vi "map to well (ROI) simple.vi"(7 "centroids in":u16[][](array[numeric])=[[65535, 65535], [65535, 65535], [57, 304], [65535, 65535], [65535, 65535], [65535, 65535], [65535, 65535], [84, 793], [150, 86], [65535, 65535], [65535, 65535], [65535, 65535], [65535, 65535], [65535, 65535], [65535, 65535], [65535, 65535], [295, 112], [65535, 65535], [65535, 65535], [65535, 65535], [65535, 65535], [65535, 65535], [65535, 65535], [313, 848], [402, 114], [65535, 65535], [65535, 65535], [65535, 65535], [65535, 65535], [65535, 65535], [65535, 65535], [65535, 65535], [65535, 65535], [65535, 65535], [65535, 65535], [65535, 65535], [65535, 65535], [65535, 65535], [65535, 65535], [65535, 65535], [65535, 65535], [65535, 65535], [65535, 65535], [65535, 65535], [65535, 65535], [65535, 65535], [562, 690], [613, 846], [733, 113], [65535, 65535], [65535, 65535], [65535, 65535], [65535, 65535], [65535, 65535], [65535, 65535], [65535, 65535], [843, 133], [65535, 65535], [65535, 65535], [65535, 65535], [65535, 65535], [65535, 65535], [65535, 65535], [65535, 65535], [880, 72], [65535, 65535], [65535, 65535], [881, 382], [65535, 65535], [65535, 65535], [65535, 65535], [65535, 65535], [989, 67], [65535, 65535], [65535, 65535], [65535, 65535], [65535, 65535], [65535, 65535], [65535, 65535], [1004, 856], [65535, 65535], [1089, 232], [65535, 65535], [65535, 65535], [65535, 65535], [65535, 65535], [65535, 65535], [1100, 861], [1253, 78], [65535, 65535], [65535, 65535], [65535, 65535], [65535, 65535], [65535, 65535], [65535, 65535], [65535, 65535]], 10 "roi data cluster":T1={[0, 0, 1280, 960], [{"Contour Type"=0, "ROI Type"=12, [70, 141, 164, 235, 270302]}, {"Contour Type"=0, "ROI Type"=12, [70, 236, 164, 330, 270302]}, {"Contour Type"=0, "ROI Type"=12, [71, 331, 165, 425, 270302]}, {"Contour Type"=0, "ROI Type"=12, [72, 426, 166, 520, 270302]}, {"Contour Type"=0, "ROI Type"=12, [72, 520, 166, 614, 270302]}, {"Contour Type"=0, "ROI Type"=12, [72, 615, 166, 709, 270302]}, {"Contour Type"=0, "ROI Type"=12, [73, 710, 167, 804, 270302]}, {"Contour Type"=0, "ROI Type"=12, [74, 805, 168, 899, 270302]}, {"Contour Type"=0, "ROI Type"=12, [165, 140, 259, 234, 270302]}, {"Contour Type"=0, "ROI Type"=12, [165, 235, 259, 329, 270302]}, {"Contour Type"=0, "ROI Type"=12, [166, 330, 260, 424, 270302]}, {"Contour Type"=0, "ROI Type"=12, [166, 425, 260, 519, 270302]}, {"Contour Type"=0, "ROI Type"=12, [167, 520, 261, 614, 270302]}, {"Contour Type"=0, "ROI Type"=12, [167, 615, 261, 709, 270302]}, {"Contour Type"=0, "ROI Type"=12, [168, 710, 262, 804, 270302]}, {"Contour Type"=0, "ROI Type"=12, [168, 805, 262, 899, 270302]}, {"Contour Type"=0, "ROI Type"=12, [260, 140, 354, 234, 270302]}, {"Contour Type"=0, "ROI Type"=12, [260, 235, 354, 329, 270302]}, {"Contour Type"=0, "ROI Type"=12, [260, 330, 354, 424, 270302]}, {"Contour Type"=0, "ROI Type"=12, [261, 425, 355, 519, 270302]}, {"Contour Type"=0, "ROI Type"=12, [262, 520, 356, 614, 270302]}, {"Contour Type"=0, "ROI Type"=12, [262, 614, 356, 708, 270302]}, {"Contour Type"=0, "ROI Type"=12, [262, 709, 356, 803, 270302]}, {"Contour Type"=0, "ROI Type"=12, [263, 804, 357, 898, 270302]}, {"Contour Type"=0, "ROI Type"=12, [354, 140, 448, 234, 270302]}, {"Contour Type"=0, "ROI Type"=12, [355, 234, 449, 328, 270302]}, {"Contour Type"=0, "ROI Type"=12, [355, 329, 449, 423, 270302]}, {"Contour Type"=0, "ROI Type"=12, [356, 424, 450, 518, 270302]}, {"Contour Type"=0, "ROI Type"=12, [356, 519, 450, 613, 270302]}, {"Contour Type"=0, "ROI Type"=12, [357, 614, 451, 708, 270302]}, {"Contour Type"=0, "ROI Type"=12, [357, 709, 451, 803, 270302]}, {"Contour Type"=0, "ROI Type"=12, [358, 804, 452, 898, 270302]}, {"Contour Type"=0, "ROI Type"=12, [449, 139, 543, 233, 270302]}, {"Contour Type"=0, "ROI Type"=12, [450, 234, 544, 328, 270302]}, {"Contour Type"=0, "ROI Type"=12, [450, 329, 544, 423, 270302]}, {"Contour Type"=0, "ROI Type"=12, [450, 424, 544, 518, 270302]}, {"Contour Type"=0, "ROI Type"=12, [451, 518, 545, 612, 270302]}, {"Contour Type"=0, "ROI Type"=12, [452, 613, 546, 707, 270302]}, {"Contour Type"=0, "ROI Type"=12, [452, 708, 546, 802, 270302]}, {"Contour Type"=0, "ROI Type"=12, [452, 803, 546, 897, 270302]}, {"Contour Type"=0, "ROI Type"=12, [544, 138, 638, 232, 270302]}, {"Contour Type"=0, "ROI Type"=12, [544, 233, 638, 327, 270302]}, {"Contour Type"=0, "ROI Type"=12, [545, 328, 639, 422, 270302]}, {"Contour Type"=0, "ROI Type"=12, [545, 423, 639, 517, 270302]}, {"Contour Type"=0, "ROI Type"=12, [546, 518, 640, 612, 270302]}, {"Contour Type"=0, "ROI Type"=12, [546, 613, 640, 707, 270302]}, {"Contour Type"=0, "ROI Type"=12, [547, 708, 641, 802, 270302]}, {"Contour Type"=0, "ROI Type"=12, [547, 803, 641, 897, 270302]}, {"Contour Type"=0, "ROI Type"=12, [638, 138, 732, 232, 270302]}, {"Contour Type"=0, "ROI Type"=12, [639, 233, 733, 327, 270302]}, {"Contour Type"=0, "ROI Type"=12, [640, 328, 734, 422, 270302]}, {"Contour Type"=0, "ROI Type"=12, [640, 423, 734, 517, 270302]}, {"Contour Type"=0, "ROI Type"=12, [640, 518, 734, 612, 270302]}, {"Contour Type"=0, "ROI Type"=12, [641, 612, 735, 706, 270302]}, {"Contour Type"=0, "ROI Type"=12, [642, 707, 736, 801, 270302]}, {"Contour Type"=0, "ROI Type"=12, [642, 802, 736, 896, 270302]}, {"Contour Type"=0, "ROI Type"=12, [733, 138, 827, 232, 270302]}, {"Contour Type"=0, "ROI Type"=12, [734, 232, 828, 326, 270302]}, {"Contour Type"=0, "ROI Type"=12, [734, 327, 828, 421, 270302]}, {"Contour Type"=0, "ROI Type"=12, [735, 422, 829, 516, 270302]}, {"Contour Type"=0, "ROI Type"=12, [735, 517, 829, 611, 270302]}, {"Contour Type"=0, "ROI Type"=12, [736, 612, 830, 706, 270302]}, {"Contour Type"=0, "ROI Type"=12, [736, 707, 830, 801, 270302]}, {"Contour Type"=0, "ROI Type"=12, [737, 802, 831, 896, 270302]}, {"Contour Type"=0, "ROI Type"=12, [828, 137, 922, 231, 270302]}, {"Contour Type"=0, "ROI Type"=12, [828, 232, 922, 326, 270302]}, {"Contour Type"=0, "ROI Type"=12, [829, 327, 923, 421, 270302]}, {"Contour Type"=0, "ROI Type"=12, [830, 422, 924, 516, 270302]}, {"Contour Type"=0, "ROI Type"=12, [830, 516, 924, 610, 270302]}, {"Contour Type"=0, "ROI Type"=12, [830, 611, 924, 705, 270302]}, {"Contour Type"=0, "ROI Type"=12, [831, 706, 925, 800, 270302]}, {"Contour Type"=0, "ROI Type"=12, [832, 801, 926, 895, 270302]}, {"Contour Type"=0, "ROI Type"=12, [923, 136, 1017, 230, 270302]}, {"Contour Type"=0, "ROI Type"=12, [923, 231, 1017, 325, 270302]}, {"Contour Type"=0, "ROI Type"=12, [924, 326, 1018, 420, 270302]}, {"Contour Type"=0, "ROI Type"=12, [924, 421, 1018, 515, 270302]}, {"Contour Type"=0, "ROI Type"=12, [925, 516, 1019, 610, 270302]}, {"Contour Type"=0, "ROI Type"=12, [925, 611, 1019, 705, 270302]}, {"Contour Type"=0, "ROI Type"=12, [926, 706, 1020, 800, 270302]}, {"Contour Type"=0, "ROI Type"=12, [926, 801, 1020, 895, 270302]}, {"Contour Type"=0, "ROI Type"=12, [1018, 136, 1112, 230, 270302]}, {"Contour Type"=0, "ROI Type"=12, [1018, 231, 1112, 325, 270302]}, {"Contour Type"=0, "ROI Type"=12, [1018, 326, 1112, 420, 270302]}, {"Contour Type"=0, "ROI Type"=12, [1019, 421, 1113, 515, 270302]}, {"Contour Type"=0, "ROI Type"=12, [1020, 516, 1114, 610, 270302]}, {"Contour Type"=0, "ROI Type"=12, [1020, 610, 1114, 704, 270302]}, {"Contour Type"=0, "ROI Type"=12, [1020, 705, 1114, 799, 270302]}, {"Contour Type"=0, "ROI Type"=12, [1021, 800, 1115, 894, 270302]}, {"Contour Type"=0, "ROI Type"=12, [1112, 136, 1206, 230, 270302]}, {"Contour Type"=0, "ROI Type"=12, [1113, 230, 1207, 324, 270302]}, {"Contour Type"=0, "ROI Type"=12, [1113, 325, 1207, 419, 270302]}, {"Contour Type"=0, "ROI Type"=12, [1114, 420, 1208, 514, 270302]}, {"Contour Type"=0, "ROI Type"=12, [1114, 515, 1208, 609, 270302]}, {"Contour Type"=0, "ROI Type"=12, [1115, 610, 1209, 704, 270302]}, {"Contour Type"=0, "ROI Type"=12, [1115, 705, 1209, 799, 270302]}, {"Contour Type"=0, "ROI Type"=12, [1116, 800, 1210, 894, 270302]}]}, 11 "Particle Measurements (Pixels)":dbl[][](array[numeric])=[[328.5, 294.5, 32.0], [330.0711111111111, 312.06666666666666, 225.0], [151.88888888888889, 401.44444444444446, 27.0], [269.3804347826087, 408.6847826086956, 92.0], [296.5652173913044, 727.3913043478261, 23.0], [271.3529411764706, 730.7205882352941, 68.0]] format="%.2f") -> (2 "centroids out":u16[][](array[numeric])=[[269, 409], [65535, 65535], [65535, 65535], [65535, 65535], [65535, 65535], [65535, 65535], [65535, 65535], [65535, 65535], [65535, 65535], [65535, 65535], [65535, 65535], [65535, 65535], [65535, 65535], [65535, 65535], [65535, 65535], [65535, 65535], [65535, 65535], [65535, 65535], [65535, 65535], [65535, 65535], [65535, 65535], [65535, 65535], [65535, 65535], [65535, 65535], [65535, 65535], [65535, 65535], [65535, 65535], [65535, 65535], [65535, 65535], [65535, 65535], [65535, 65535], [65535, 65535], [65535, 65535], [65535, 65535], [65535, 65535], [65535, 65535], [65535, 65535], [65535, 65535], [65535, 65535], [65535, 65535], [65535, 65535], [65535, 65535], [65535, 65535], [65535, 65535], [65535, 65535], [65535, 65535], [65535, 65535], [65535, 65535], [65535, 65535], [65535, 65535], [65535, 65535], [65535, 65535], [65535, 65535], [65535, 65535], [65535, 65535], [65535, 65535], [65535, 65535], [65535, 65535], [65535, 65535], [65535, 65535], [65535, 65535], [65535, 65535], [65535, 65535], [65535, 65535], [65535, 65535], [65535, 65535], [65535, 65535], [65535, 65535], [65535, 65535], [65535, 65535], [65535, 65535], [65535, 65535], [65535, 65535], [65535, 65535], [65535, 65535], [65535, 65535], [65535, 65535], [65535, 65535], [65535, 65535], [65535, 65535], [65535, 65535], [65535, 65535], [65535, 65535], [65535, 65535], [65535, 65535], [65535, 65535], [65535, 65535], [65535, 65535], [65535, 65535], [65535, 65535], [65535, 65535], [65535, 65535], [65535, 65535], [65535, 65535], [65535, 65535], [65535, 65535]], 3 "roi total motion":u16[](array[numeric])=[467, 0, 0, 0, 0, 0, 0, 0, 0, 0, 0, 0, 0, 0, 0, 0, 0, 0, 0, 0, 0, 0, 0, 0, 0, 0, 0, 0, 0, 0, 0, 0, 0, 0, 0, 0, 0, 0, 0, 0, 0, 0, 0, 0, 0, 0, 0, 0, 0, 0, 0, 0, 0, 0, 0, 0, 0, 0, 0, 0, 0, 0, 0, 0, 0, 0, 0, 0, 0, 0, 0, 0, 0, 0, 0, 0, 0, 0, 0, 0, 0, 0, 0, 0, 0, 0, 0, 0, 0, 0, 0, 0, 0, 0, 0, 0])   [LabVIEW 2013]
panel:
  out "fish detected":bool[](array[boolean])=[TRUE, FALSE, FALSE, FALSE, FALSE, FALSE, FALSE, FALSE, FALSE, FALSE, FALSE, FALSE, FALSE, FALSE, FALSE, FALSE, FALSE, FALSE, FALSE, FALSE, FALSE, FALSE, FALSE, FALSE, FALSE, FALSE, FALSE, FALSE, FALSE, FALSE, FALSE, FALSE, FALSE, FALSE, FALSE, FALSE, FALSE, FALSE, FALSE, FALSE, FALSE, FALSE, FALSE, FALSE, FALSE, FALSE, FALSE, FALSE, FALSE, FALSE, FALSE, FALSE, FALSE, FALSE, FALSE, FALSE, FALSE, FALSE, FALSE, FALSE, FALSE, FALSE, FALSE, FALSE, FALSE, FALSE, FALSE, FALSE, FALSE, FALSE, FALSE, FALSE, FALSE, FALSE, FALSE, FALSE, FALSE, FALSE, FALSE, FALSE, FALSE, FALSE, FALSE, FALSE, FALSE, FALSE, FALSE, FALSE, FALSE, FALSE, FALSE, FALSE, FALSE, FALSE, FALSE, FALSE]
  out "multifish":bool[](array[boolean])=[TRUE, FALSE, FALSE, FALSE, FALSE, FALSE, FALSE, FALSE, FALSE, FALSE, FALSE, FALSE, FALSE, FALSE, FALSE, FALSE, FALSE, FALSE, FALSE, FALSE, FALSE, FALSE, FALSE, FALSE, FALSE, FALSE, FALSE, FALSE, FALSE, FALSE, FALSE, FALSE, FALSE, FALSE, FALSE, FALSE, FALSE, FALSE, FALSE, FALSE, FALSE, FALSE, FALSE, FALSE, FALSE, FALSE, FALSE, FALSE, FALSE, FALSE, FALSE, FALSE, FALSE, FALSE, FALSE, FALSE, FALSE, FALSE, FALSE, FALSE, FALSE, FALSE, FALSE, FALSE, FALSE, FALSE, FALSE, FALSE, FALSE, FALSE, FALSE, FALSE, FALSE, FALSE, FALSE, FALSE, FALSE, FALSE, FALSE, FALSE, FALSE, FALSE, FALSE, FALSE, FALSE, FALSE, FALSE, FALSE, FALSE, FALSE, FALSE, FALSE, FALSE, FALSE, FALSE, FALSE]
  in  "lower limit":dbl=25.0
  in  "upper limit":dbl=2000.0
  out "Waveform Graph":u16[](graph)=[467, 0, 0, 0, 0, 0, 0, 0, 0, 0, 0, 0, 0, 0, 0, 0, 0, 0, 0, 0, 0, 0, 0, 0, 0, 0, 0, 0, 0, 0, 0, 0, 0, 0, 0, 0, 0, 0, 0, 0, 0, 0, 0, 0, 0, 0, 0, 0, 0, 0, 0, 0, 0, 0, 0, 0, 0, 0, 0, 0, 0, 0, 0, 0, 0, 0, 0, 0, 0, 0, 0, 0, 0, 0, 0, 0, 0, 0, 0, 0, 0, 0, 0, 0, 0, 0, 0, 0, 0, 0, 0, 0, 0, 0, 0, 0]
  out "well number":dbl
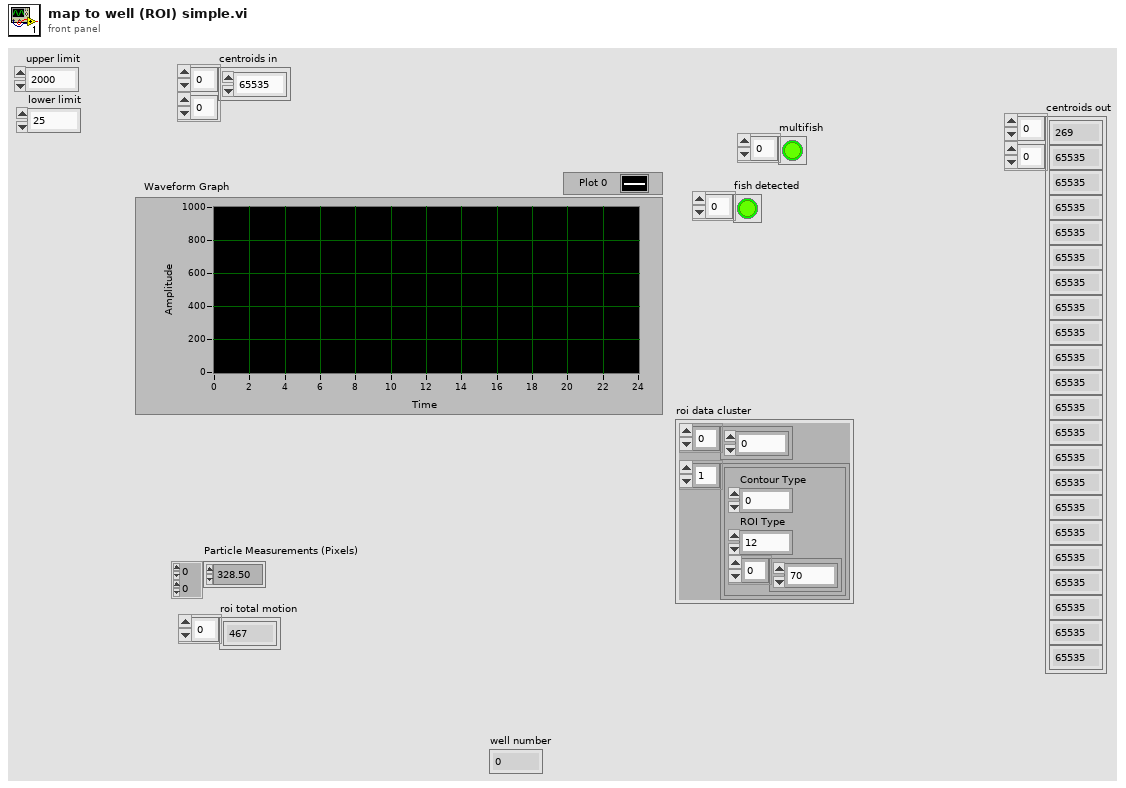
[diagram p1: front panel]
types:
  T1 = cluster{i32[], cluster{"Contour Type":u32, "ROI Type":u32, i32[]}[]}
  T2 = cluster{"Contour Type":u32, "ROI Type":u32, i32[]}[]
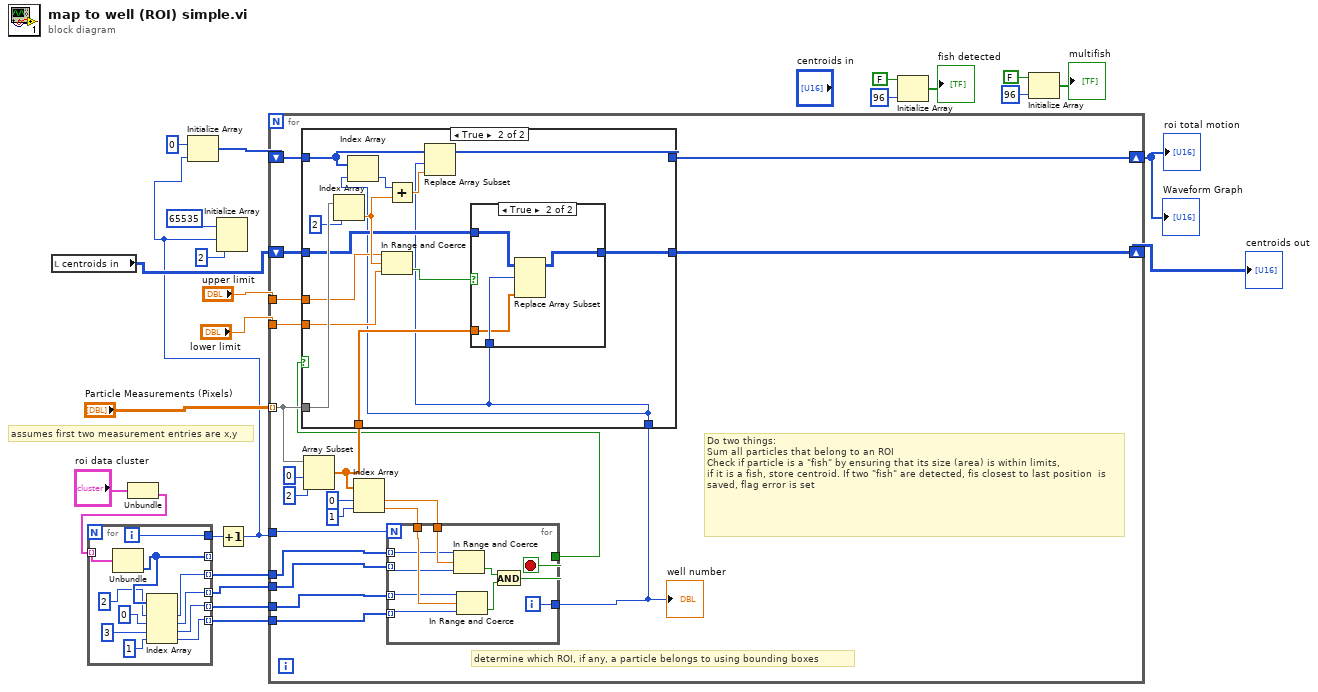
[diagram p0: block diagram]
diagram:
  # "assumes first two measurement entries are x,y"
  n1 = local read "centroids in"() -> (w4:u16[][])
  n2 = Unbundle("roi data cluster") -> (w9:T2)  [unwired: 1 out]
  n3 = for {
    tunnel: w9 -> [w35] mode=indexing
    tunnel: [w30] -> _ mode=indexing
    tunnel: [w34] -> w2
    tunnel: [w28] -> w8 mode=indexing
    tunnel: [w27] -> w7 mode=indexing
    tunnel: [w26] -> w6 mode=indexing
    tunnel: [w25] -> w5 mode=indexing
    i -> [w34]
    n4 = Unbundle(w35) -> (w30:i32[])  [unwired: 2 out]
    n5 = Index Array(array=w30, index #1=2 ("index"), index #2=0 ("index"), index #3=3 ("index"), index #4=1 ("index")) -> (element #1=w28:i32, element #2=w27:i32, element #3=w26:i32, element #4=w25:i32)
  }
  n6 = Increment(x=w2) -> (x+1=w1:i32)
  n7 = Initialize Array(u16 0 ("element"), w1) -> (w22:u16[])
  n8 = Initialize Array(u16 65535 ("element"), w1, 2 ("dimension size")) -> ()  [unwired: 1 out]
  n9 = for {
    tunnel: "Particle Measurements (Pixels)" -> [w55] mode=indexing
    shift-right: [w53] -> w21
    shift-left: w22 -> [w54]
    shift-right: [w49] -> w3
    shift-left: w4 -> [w50]
    tunnel: "upper limit" -> [w52]
    tunnel: "lower limit" -> [w51]
    tunnel: w1 -> [w44]
    tunnel: w8 -> [w39]
    tunnel: w7 -> [w38]
    tunnel: w6 -> [w37]
    tunnel: w5 -> [w36]
    # "Do two things: \nSum all particles that belong to an ROI\nCheck if particle is a \"fish\" by ensuring that its size (area) is within limits,\nif it is a fish, store centroid. If two \"fish\" are detected, fis closest to last position  is saved, flag error is set"
    # "determine which ROI, if any, a particle belongs to using bounding boxes"
    n10 = Array Subset(array=w55, index=0, length=2 ("index")) -> (w47:dbl[])
    n11 = Index Array(array=w47, index #1=0 ("index"), index #2=1 ("index")) -> (element #1=w43:dbl, element #2=w42:dbl)
    n12 = for {
      N: w44 -> [_]
      tunnel: w43 -> [w87]
      tunnel: w42 -> [w86]
      tunnel: [w83] -> w41
      tunnel: [w82] -> w40
      tunnel: w39 -> [w81] mode=indexing
      tunnel: w38 -> [w80] mode=indexing
      tunnel: w37 -> [w79] mode=indexing
      tunnel: w36 -> [w78] mode=indexing
      i -> [w83]
      stop <- w82 stop-if-true
      n13 = In Range and Coerce(upper limit=w81, x=w87, lower limit=w80) -> (In Range?=w85:bool)  [unwired: 1 out]
      n14 = In Range and Coerce(upper limit=w79, x=w86, lower limit=w78) -> (In Range?=w84:bool)  [unwired: 1 out]
      n15 = And(x=w85, y=w84) -> (x .and. y?=w82:bool)
    }
    "well number" <- w41
    n16 = case shown="True" w40 {
      tunnel: w55 -> [_ w71]
      tunnel: w54 -> [w58 w69]
      tunnel: [w58 w67] -> w53
      tunnel: w52 -> [_ w65]
      tunnel: w51 -> [_ w64]
      tunnel: w50 -> [w57 w62]
      tunnel: [w57 w61] -> w49
      tunnel: w47 -> [_ w60]
      tunnel: w41 -> [_ w59]
      frame False {
      }
      frame True {
        n17 = Index Array(array=w71, index=2) -> (element=w66:dbl)
        n18 = Index Array(array=w69, index=w59) -> (element=w72:u16)
        n19 = In Range and Coerce(upper limit=w65, x=w66, lower limit=w64) -> (In Range?=w63:bool)  [unwired: 1 out]
        n20 = Add(x=w72, y=w66) -> (x+y=w68:dbl)
        n21 = Replace Array Subset(array=w69, new element=w68, index=w59) -> (w67:u16[])
        n22 = case shown="True" w63 {
          tunnel: w62 -> [w73 w77]
          tunnel: [w73 w74] -> w61
          tunnel: w59 -> [_ w76]
          tunnel: w60 -> [_ w75]
          frame False {
          }
          frame True {
            n23 = Replace Array Subset(array=w77, new element=w75, index (row)=w76) -> (w74:u16[][])  [unwired: 1 in]
          }
        }
      }
    }
  }
  "roi total motion" <- w21
  "Waveform Graph" <- w21
  "centroids out" <- w3
  n24 = Initialize Array(FALSE, 96 ("dimension size")) -> (→"fish detected":bool[])
  n25 = Initialize Array(FALSE, 96 ("dimension size")) -> (→"multifish":bool[])
